vi "Create Parameterized Suite.vi"(8 "error in (no error)":errorcluster) -> (0 "error out":errorcluster, 3 "Parameterized Test Suite":refnum<class "Parameterized Test Suite.lvclass">)   [LabVIEW 2020, in "Parameterized Test Suite.lvclass"]
uses:
  Parameterized Test Suite.lvclass
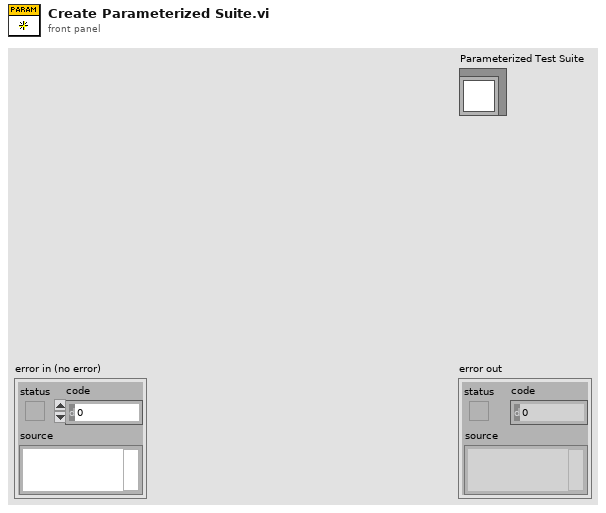
[diagram p1: front panel]
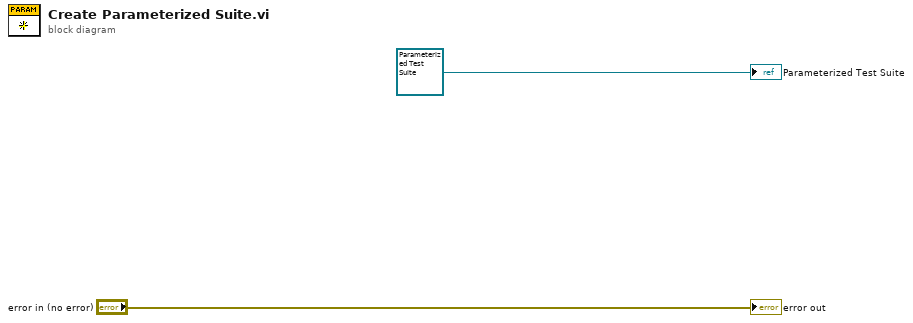
[diagram p0: block diagram]
diagram:
  "error out" <- "error in (no error)"
  "Parameterized Test Suite" <- refnum<class "Parameterized Test Suite.lvclass"> refnum ("Parameterized Test Suite")
